vi "Emballage_BDD_RESULT_S1220009_bdd.vi"(8 "error in (no error)":errorcluster, 11 "SN_PRODUIT":string) -> (0 "error out":errorcluster, 2 "dernière_donnée":string[](array[string]), 3 "result":bool)   [LabVIEW 2020]
uses:
  Modules/FS/60_FS_Controles/60_FS_SetGet.ctl
  <vilib>/addons/database/Connection.llb/DB Tools Open Connec (Path).vi
  <vilib>/addons/database/Connection.llb/Conn Execute.vi
  <vilib>/addons/database/Recordset.llb/Rec Fetch Recordset Data (R).vi
  <vilib>/addons/database/Recordset.llb/Rec Destroy - Connection.vi
  <vilib>/addons/database/NI_Database_API.lvlib
panel:
  out "data":string[][](array[string])
  out "données":string[][](array[string])
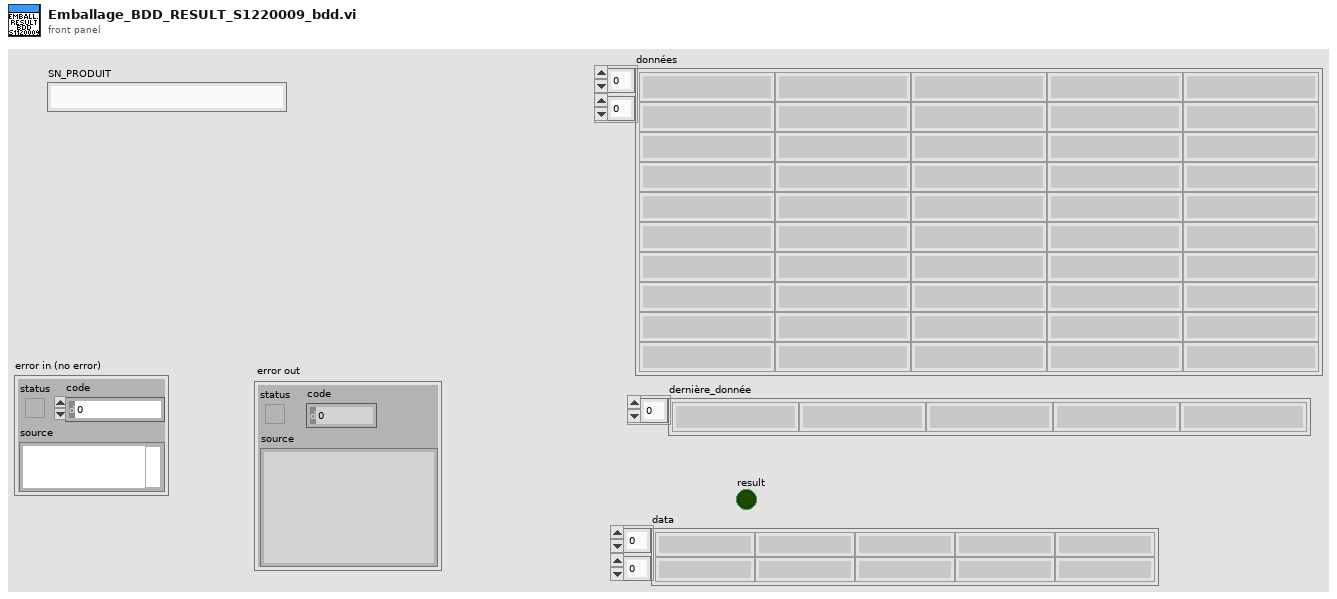
[diagram p1: front panel]
types:
  T1 = typedef "60_FS_SetGet.ctl" = enum16{"set", "get"}
  T2 = typedef "60_FS_CLT_Chemins.ctl" = cluster{"Racine_local":path, "Racine_reseau":path, "Racine_Support_Application":path, "Fichier_Journalisation":path, "Connexion_BDD_VSX":path, "Connexion_BDD_PLZ":path}
  T3 = typedef "NI_Database_API.lvlib/Conn ObjectReference.ctl" = refnum<k1>
  T4 = typedef "NI_Database_API.lvlib/Rec ObjectReference.ctl" = refnum<k1>
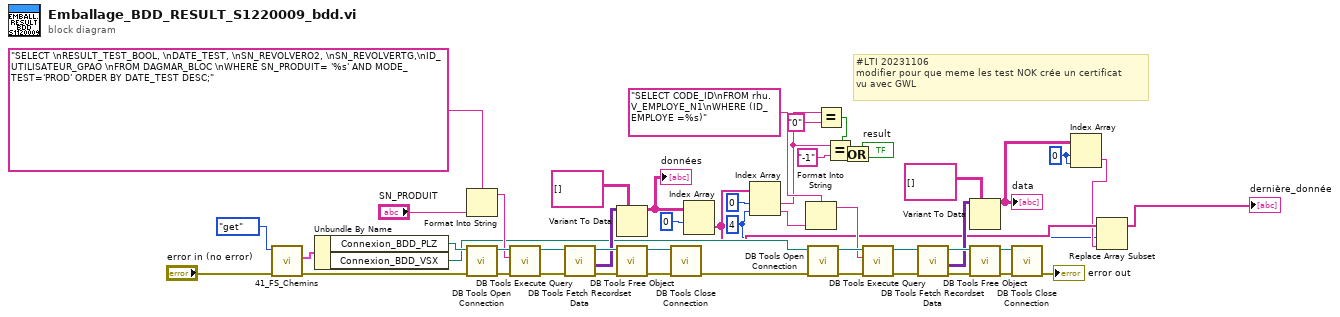
[diagram p0: block diagram]
diagram:
  w7 = 0 ("index (row)")
  w5 = 4 ("index")
  # "#LTI 20231106\nmodifier pour que meme les test NOK crée un certificat\nvu avec GWL"
  n1 = call "41_FS_Chemins.vi"("error in (no error)"="error in (no error)", "SetGet"=60_FS_SetGet."get") -> ("error out"=w41:errorcluster, "CLT_Chemins_out"=w48:T2)  [unwired: 8 in]
  n2 = Unbundle By Name(w48) -> ("Connexion_BDD_PLZ"=w42:path, "Connexion_BDD_VSX"=w18:path)
  n3 = Format Into String(format string="SELECT \nRESULT_TEST_BOOL, \nDATE_TEST, \nSN_REVOLVERO2, \nSN_REVOLVERTG,\nID_UTILISATEUR_GPAO \nFROM DAGMAR_BLOC \nWHERE SN_PRODUIT= '%s' AND MODE_TEST='PROD' ORDER BY DATE_TEST DESC;" ("SQL query"), "SN_PRODUIT") -> (resulting string=w33:string)  [unwired: 2 in, 1 out]
  n4 = call-poly <vilib>:"DB Tools Open Connection.vi"("error in (no error)"=w41, "connection information"=w42) -> ("error out"=w46:errorcluster, "connection reference"=w40:T3)  [unwired: 6 in]
  n5 = call-poly <vilib>:"DB Tools Execute Query.vi"("error in (no error)"=w46, "SQL query"=w33, "connection reference"=w40) -> ("error out"=w43:errorcluster, "recordset reference"=w39:T4)  [unwired: 5 in]
  n6 = call-poly <vilib>:"DB Tools Fetch Recordset Data.vi"("error in (no error)"=w43, "recordset reference"=w39) -> ("error out"=w44:errorcluster, "recordset data"=w36:variant[][], "recordset reference out"=w38:T4)  [unwired: 3 in]
  n7 = Variant To Data(type=string[][] [] ("Liste des champs à lire 2"), Variant=w36) -> (data=w31:string[][])  [unwired: 1 in, 1 out]
  "données" <- w31
  n8 = call-poly <vilib>:"DB Tools Free Object.vi"("error in (no error)"=w44, "recordset reference"=w38) -> ("error out"=w45:errorcluster, "connection reference"=w37:T3)  [unwired: 8 in]
  n9 = call <vilib>:"DB Tools Close Connection.vi"("error in (no error)"=w45, "connection reference"=w37) -> ("error out"=w17:errorcluster)  [unwired: 5 in]
  n10 = Index Array(array=w31, index (row)=0 ("indice (ligne)")) -> (element=w9:string[])  [unwired: 1 in]
  n11 = Index Array(array=w9, index #1=0 ("indice"), index #2=w5) -> (element #1=w3:string, element #2=w14:string)
  n12 = Format Into String(format string="SELECT CODE_ID\nFROM rhu.V_EMPLOYE_N1\nWHERE (ID_EMPLOYE =%s)" ("SQL query"), w14) -> (resulting string=w13:string)  [unwired: 2 in, 1 out]
  n13 = call-poly <vilib>:"DB Tools Open Connection.vi"("error in (no error)"=w17, "connection information"=w18) -> ("error out"=w19:errorcluster, "connection reference"=w23:T3)  [unwired: 6 in]
  n14 = Equal?(x=w3, y="0") -> (x = y?=w1:bool)
  n15 = Equal?(x=w3, y="-1") -> (x = y?=w28:bool)
  n16 = Or(x=w28, y=w1) -> (x .or. y?=→"result":bool)
  n17 = call-poly <vilib>:"DB Tools Execute Query.vi"("error in (no error)"=w19, "SQL query"=w13, "connection reference"=w23) -> ("error out"=w22:errorcluster, "recordset reference"=w24:T4)  [unwired: 5 in]
  n18 = call-poly <vilib>:"DB Tools Fetch Recordset Data.vi"("error in (no error)"=w22, "recordset reference"=w24) -> ("error out"=w21:errorcluster, "recordset data"=w11:variant[][], "recordset reference out"=w25:T4)  [unwired: 3 in]
  n19 = Variant To Data(type=string[][] [] ("Liste des champs à lire 2"), Variant=w11) -> (data=w8:string[][])  [unwired: 1 in, 1 out]
  "data" <- w8
  n20 = call-poly <vilib>:"DB Tools Free Object.vi"("error in (no error)"=w21, "recordset reference"=w25) -> ("error out"=w20:errorcluster, "connection reference"=w26:T3)  [unwired: 8 in]
  n21 = call <vilib>:"DB Tools Close Connection.vi"("error in (no error)"=w20, "connection reference"=w26) -> ("error out"=→"error out":errorcluster)  [unwired: 5 in]
  n22 = Index Array(array=w8, index (row)=w7, index (col)=w7) -> (element=w6:string)
  n23 = Replace Array Subset(array=w9, new element=w6, index=w5) -> (→"dernière_donnée":string[])
